vi "Mask Write Register Response.vi"(8 "error in (no error)":errorcluster, 10 "Modbus data unit in":refnum<class "Modbus Data Unit (PDU).lvclass">) -> (0 "error out":errorcluster, 1 "AND mask":u16, 2 "address":u16, 5 "OR mask":u16)   [LabVIEW 2020, in "SubVIs.lvlib" / "Master Function Definition.lvlib"]
doc: "Decodes the response for the masked write single register function."
uses:
  <vilib>/Modbus/subvis/Data and Functions/Master Function Definition/Master Function Definition.lvlib
  <vilib>/Modbus/subvis/Modbus Data Unit (PDU)/Modbus Data Unit (PDU).lvclass
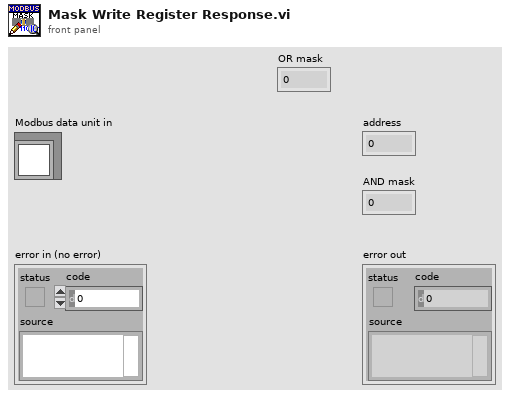
[diagram p1: front panel]
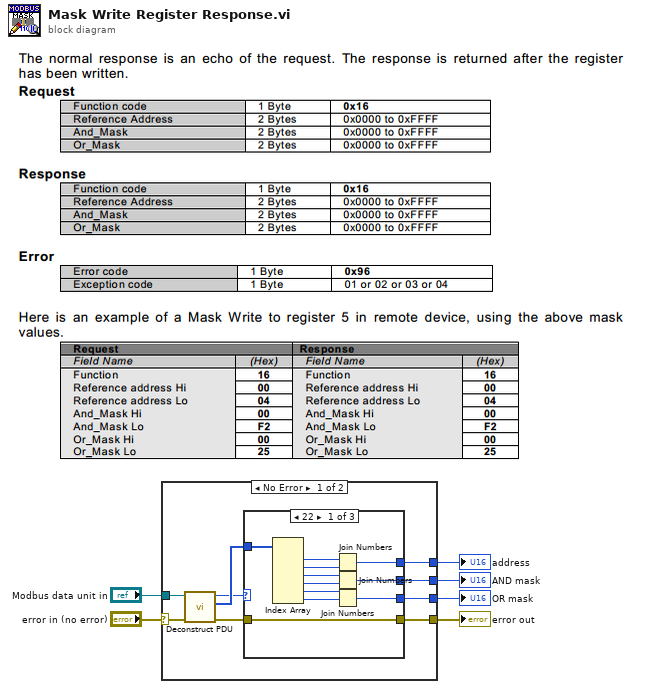
[diagram p0: block diagram]
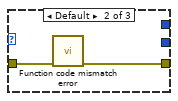
[diagram p2: hidden frame]
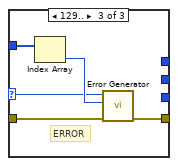
[diagram p3: hidden frame]
diagram:
  n1 = case shown="No Error" "error in (no error)" {
    selector: "error in (no error)" -> [w7 w34]
    tunnel: [w15 w34] -> w6
    tunnel: "Modbus data unit in" -> [w13 _]
    tunnel: [w11 _] -> w4
    tunnel: [w10 _] -> w3
    tunnel: [w8 _] -> w2
    frame No Error {
      n2 = call <vilib>:"Deconstruct PDU.vi"("error in (no error)"=w7, "Modbus data unit in"=w13) -> ("error out"=w12:errorcluster, "data"=w14:u8[], "function"=w9:u8)  [unwired: 7 in]
      n3 = case shown="22" w9 {
        selector: w9 -> [_ _ w29]
        tunnel: w12 -> [w25 w27 w30]
        tunnel: w14 -> [w26 _ w33]
        tunnel: [w25 w28 w32] -> w15
        tunnel: [w24 _ _] -> w11
        tunnel: [w23 _ _] -> w10
        tunnel: [w16 _ _] -> w8
        frame 22 {
          n4 = Index Array(array=w26) -> (element #1=w22:u8, element #2=w21:u8, element #3=w20:u8, element #4=w19:u8, element #5=w18:u8, element #6=w17:u8)  [unwired: 6 in]
          n5 = Join Numbers(hi=w22, lo=w21) -> ((hi.lo)=w24:u16)
          n6 = Join Numbers(hi=w20, lo=w19) -> ((hi.lo)=w23:u16)
          n7 = Join Numbers(hi=w18, lo=w17) -> ((hi.lo)=w16:u16)
        }
        frame Default {
          n8 = call <vilib>:"Function code mismatch error.vi"("error in (no error)"=w27) -> ("error out"=w28:errorcluster)  [unwired: 10 in]
        }
        frame 129.. {
          # "ERROR"
          n9 = Index Array(array=w33) -> (element=w31:u8)  [unwired: 1 in]
          n10 = call <vilib>:"Error Generator.vi"("error in (no error)"=w30, "data return (error code)"=w31, "function return"=w29) -> ("error out"=w32:errorcluster)  [unwired: 8 in]
        }
      }
    }
    frame Error {
    }
  }
  "error out" <- w6
  "address" <- w4
  "AND mask" <- w3
  "OR mask" <- w2
